vi "Get Kaelus System Directory.vi"(5 "Base Directory (Kaelus)":enum16{"Kaelus", "Summitek"}(ring), 7 "create directory if not found? (T)":bool=TRUE, 10 "Relative Directory Path (Directory only please)":string, 11 "Directory Type (Public App Data)":T1=7 items=["User Home"=0, "User Desktop"=1, "User Documents"=2, "User Application Data"=3, "User Preferences"=4, "User Temporary"=5, "Public Documents"=6, "Public Application Data"=7, "Public Preferences"=8, "Public Cache"=13, "System Core Libraries"=9, "System Installed Libraries"=10, "Application Files"=11, "Boot Volume Root"=12]) -> (2 "Summitek ProgramData + Relative":path)   [LabVIEW 2011]
uses:
  <vilib>/Utility/sysdir.llb/System Directory Type.ctl
  OpenG EXT/file/file.llb/Append Path to Root if Relative - Scalar__ogtk.vi
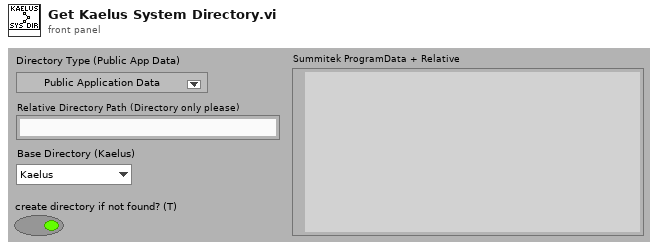
[diagram p1: front panel]
types:
  T1 = typedef "System Directory Type.ctl" = i32
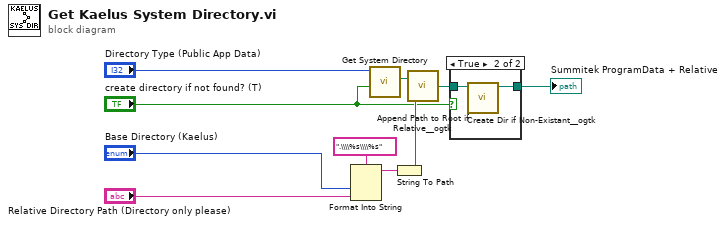
[diagram p0: block diagram]
diagram:
  n1 = Format Into String(format string=".\\\\%s\\\\%s" ("name or relative path"), "Base Directory (Kaelus)", "Relative Directory Path (Directory only please)") -> (resulting string=w7:string)  [unwired: 2 in, 1 out]
  n2 = call <vilib>:"Get System Directory.vi"("create directory if not found? (F)"="create directory if not found? (T)", "system directory type"="Directory Type (Public App Data)") -> ("system directory"=w10:path)  [unwired: 9 in]
  n3 = String To Path(string=w7) -> (path=w6:path)
  n4 = call-poly "Append Path to Root if Relative__ogtk.vi"("Absolute or Relative Path"=w6, "Root Path"=w10) -> ("Absolute or Appended Path"=w5:path)
  n5 = case shown="True" "create directory if not found? (T)" {
    tunnel: w5 -> [w11 w13]
    tunnel: [w11 w12] -> w3
    frame False {
    }
    frame True {
      n6 = call "Create Dir if Non-Existant__ogtk.vi"("Directory Path"=w13) -> ("dup Directory Path"=w12:path)  [unwired: 8 in, 2 out]
    }
  }
  "Summitek ProgramData + Relative" <- w3
